vi "DHE_SetModRef.vi"(2 "DHE_ModRef":refnum<vi>) -> ()   [LabVIEW 2016]
uses:
  DHE_GBLDriverVariables.vi
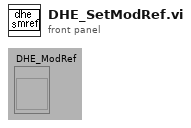
[diagram p1: front panel]
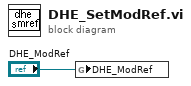
[diagram p0: block diagram]
diagram:
  n1 = global write "DHE_GBLDriverVariables.vi" "DHE_ModRef"("DHE_ModRef") -> ()
